vi "imaqdx open camera.vi"(8 "error in (no error)":errorcluster, 10 "Config File":path, 11 "identifier":string) -> (0 "error out":errorcluster, 3 "Session Out":T1)   [LabVIEW 2022 SP3, in "Vision.lvlib"]
uses:
  Vision.lvlib
  <vilib>/userDefined/High Color/IMAQdx.ctl
  <vilib>/vision/driver/NI_Vision_Acquisition_Software.lvlib
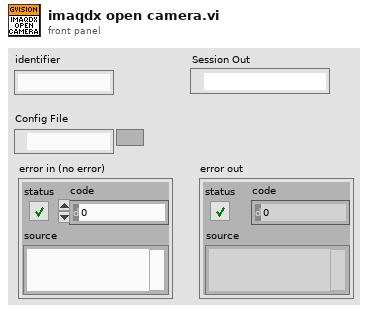
[diagram p1: front panel]
types:
  T1 = typedef "IMAQdx.ctl" = refnum<k21>
  T2 = cluster{"Type":u32, "Version":u32, "Flags":u32, "SerialNumberHigh":u32, "SerialNumberLow":u32, "BusType":u32, "InterfaceName":string, "VendorName":string, "ModelName":string, "CameraFileName":string, "CameraAttributeURL":string}[]
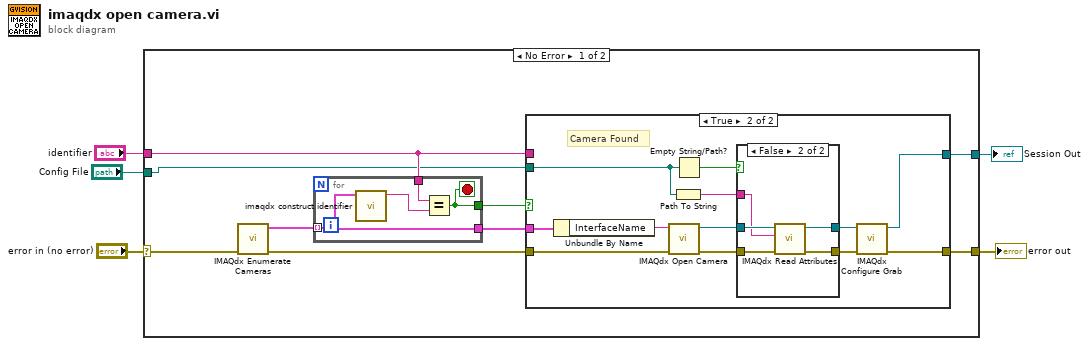
[diagram p0: block diagram]
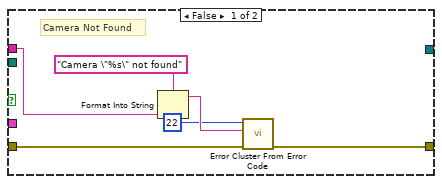
[diagram p2: hidden frame]
diagram:
  n1 = case shown="No Error" "error in (no error)" {
    selector: "error in (no error)" -> [w14 w44]
    tunnel: [w10 w44] -> w4
    tunnel: "identifier" -> [w9 _]
    tunnel: "Config File" -> [w6 _]
    tunnel: [w7 _] -> w1
    frame No Error {
      n2 = call <vilib>:"IMAQdx Enumerate Cameras.vi"("error in"=w14) -> ("error out"=w11:errorcluster, "Camera Information Array"=w13:T2)  [unwired: 9 in]
      n3 = for {
        tunnel: w13 -> [w41] mode=indexing
        tunnel: w9 -> [w43]
        tunnel: [w41] -> w8
        tunnel: [w40] -> w12
        stop <- w40 stop-if-true
        n4 = call "imaqdx construct identifier.vi"("Camera Information"=w41) -> ("resulting string"=w42:string)  [unwired: 10 in]
        n5 = Equal?(x=w43, y=w42) -> (x = y?=w40:bool)
      }
      n6 = case shown="True" w12 {
        tunnel: w11 -> [w20 w32]
        tunnel: [w19 w25] -> w10
        tunnel: w9 -> [w17 _]
        tunnel: w8 -> [_ w31]
        tunnel: [_ w24] -> w7
        tunnel: w6 -> [_ w22]
        frame False {
          # "Camera Not Found"
          n7 = Format Into String(format string="Camera \"%s\" not found", w17) -> (resulting string=w16:string)  [unwired: 2 in, 1 out]
          n8 = call <vilib>:"Error Cluster From Error Code.vi"("error in (no error)"=w20, "error message (\"\")"=w16, "error code (0)"=22) -> ("error out"=w19:errorcluster)  [unwired: 6 in]
        }
        frame True {
          # "Camera Found"
          n9 = Unbundle By Name(w31) -> ("InterfaceName"=w30:string)
          n10 = call <vilib>:"IMAQdx Open Camera.vi"("error in"=w32, "Session In"=w30) -> ("error out"=w28:errorcluster, "Session Out"=w29:T1)  [unwired: 8 in]
          n11 = Path To String(path=w22) -> (string=w21:string)
          n12 = Empty String/Path?(string/path=w22) -> (empty?=w23:bool)
          n13 = case shown="False" w23 {
            tunnel: w29 -> [w34 w39]
            tunnel: w28 -> [w33 w38]
            tunnel: [w34 w37] -> w27
            tunnel: [w33 w36] -> w26
            tunnel: w21 -> [_ w35]
            frame True {
            }
            frame False {
              n14 = call <vilib>:"IMAQdx Read Attributes.vi"("error in"=w38, "Filename"=w35, "Session In"=w39) -> ("error out"=w36:errorcluster, "Session Out"=w37:T1)  [unwired: 7 in]
            }
          }
          n15 = call <vilib>:"IMAQdx Configure Grab.vi"("error in"=w26, "Session In"=w27) -> ("error out"=w25:errorcluster, "Session Out"=w24:T1)  [unwired: 8 in]
        }
      }
    }
    frame Error {
    }
  }
  "error out" <- w4
  "Session Out" <- w1
